vi "Printing Loop XYZ.vi"(11 "Stage Actor in":refnum<class "Stage.lvclass">) -> (3 "data value reference":refnum<data-value>)   [LabVIEW 2018, in "Stage Actor.lvlib" / "Stage.lvclass"]
uses:
  Stage.lvclass
  C:/Program Files/National Instruments/LabVIEW 2018/vi.lib/MGI/Panel Manager/Panel Actor/Panel Actor/Panel Actor.lvclass
  C:/Program Files/National Instruments/LabVIEW 2018/vi.lib/ActorFramework/Actor/Actor.lvclass
  Print Type Def.ctl
  <vilib>/ActorFramework/Actor/Actor.lvclass/Actor.ctl
  Stage.lvclass/Stage.ctl
  ADM/Main Messages/Set Flow Msg/Set Flow Msg.lvclass/Set Flow Msg.ctl
  <vilib>/ActorFramework/Message Enqueuer/Message Enqueuer.lvclass/Message Enqueuer.ctl
  ea4cf82d-fce5-4455-9177-557e4ebb6024.vi
  <vilib>/ActorFramework/Message Enqueuer/Enqueue.vi
  ADM/Main Messages/Set Flow Msg/Set Flow Msg.lvclass
  C:/Program Files/National Instruments/LabVIEW 2018/vi.lib/ActorFramework/Message/Message.lvclass
  Stage Messages/End Print Msg/End Print Msg.lvclass
  <vilib>/ActorFramework/Message Priority Queue/Priority Enqueue.vi
  <vilib>/MGI/Panel Manager/Panel Actor/Panel Actor/Panel Actor.lvclass
  Stage Actor.lvlib
  <instrlib>/Zaber A Series/Zaber A Series.lvlib
  <vilib>/ActorFramework/Actor/Actor.lvclass
panel:
  in  "Print Cancelled":bool
  in  "Stop":bool
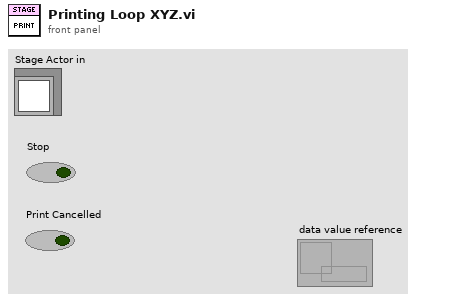
[diagram p1: front panel]
types:
  T1 = typedef "Stage Actor.lvlib/Print Type Def.ctl" = enum16{"Wait for Command", "Print Line", "End Print", "End"}
  T2 = cluster{"Current Tool":i16, "Speed":dbl, "Feeder State":bool, "Z":dbl, "XY":dbl[], "Theta Phi":dbl[]}
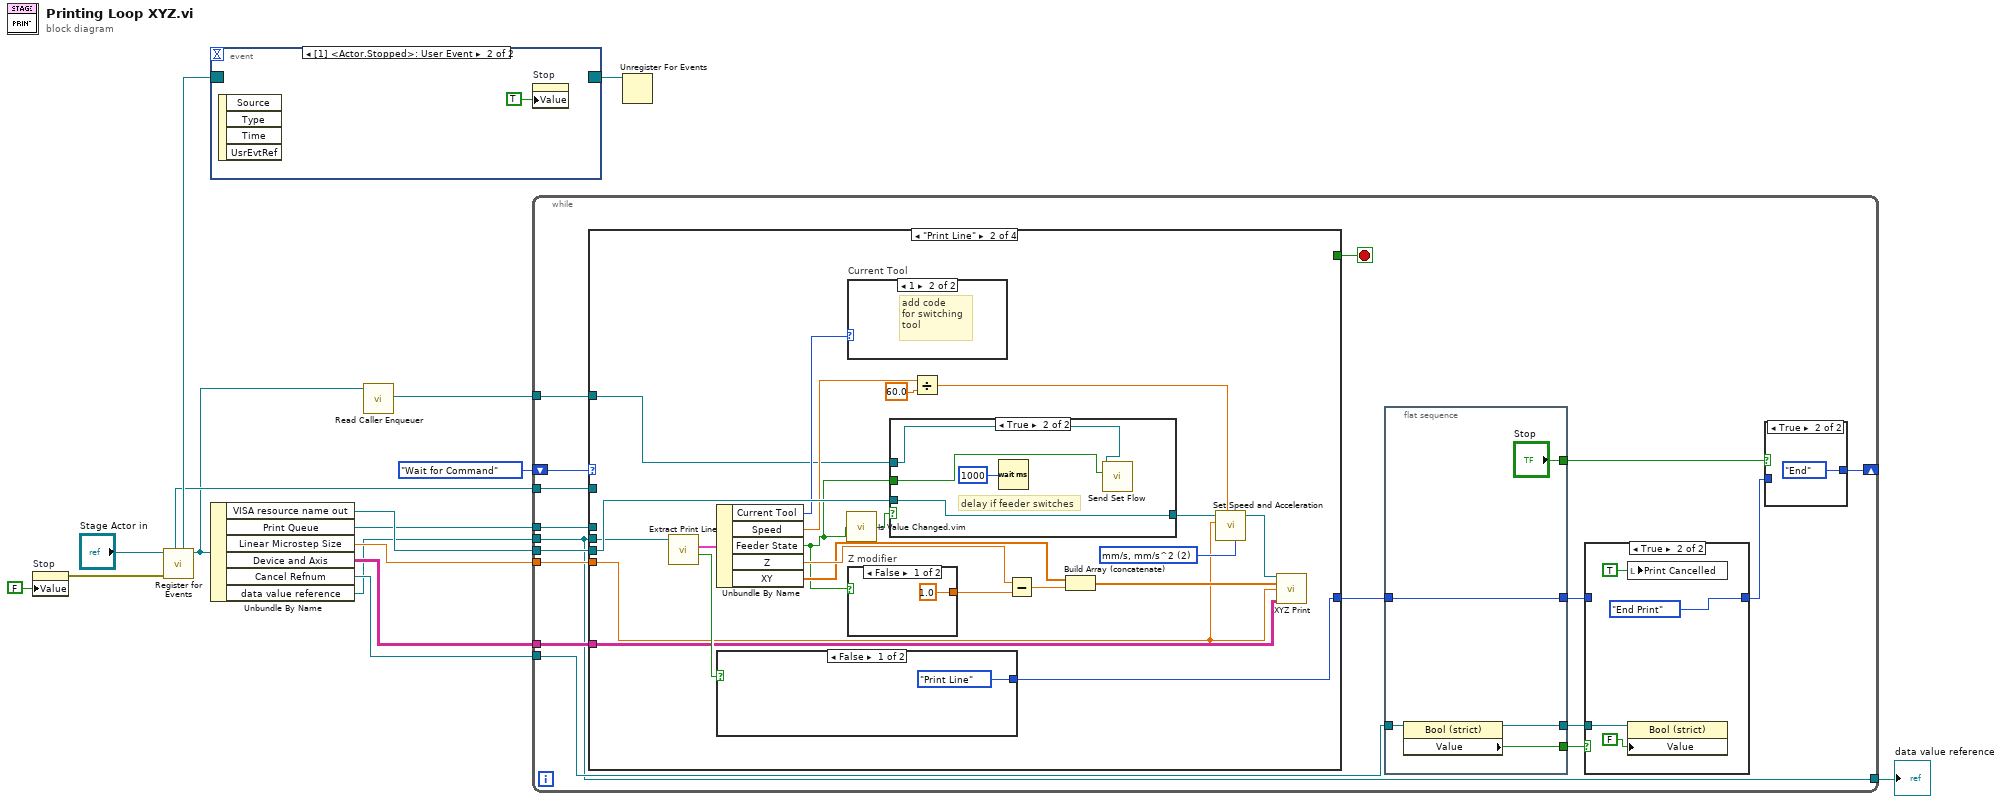
[diagram p0: block diagram]
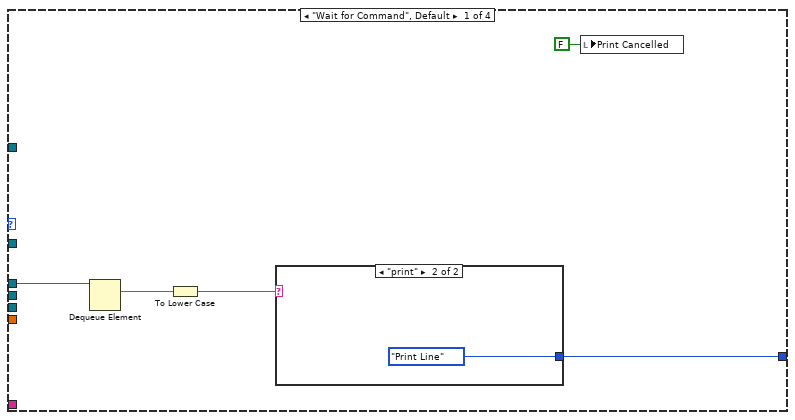
[diagram p4: hidden frame]
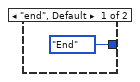
[diagram p5: hidden frame]
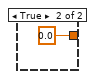
[diagram p6: hidden frame]
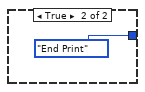
[diagram p7: hidden frame]
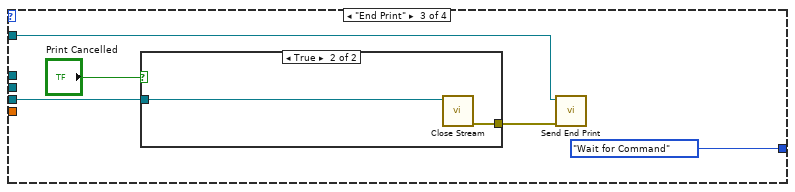
[diagram p10: hidden frame]
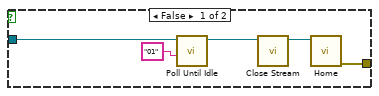
[diagram p11: hidden frame]
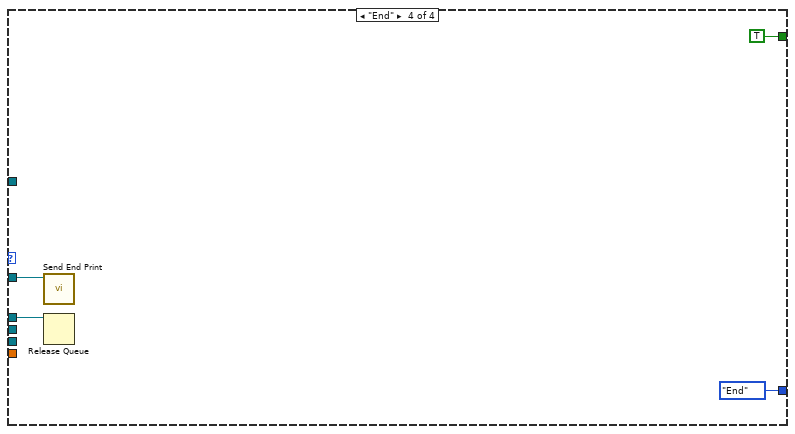
[diagram p12: hidden frame]
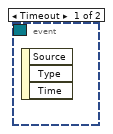
[diagram p13: hidden frame]
diagram:
  n1 = property on="Stop" class="Bool (strict)"("Value"=FALSE ("Stop")) -> (error out=w15:errorcluster)  [unwired: 2 in, 1 out]
  n2 = call <vilib>:"Register for Events.vi"("Error In"=w15, "Panel Actor in"="Stage Actor in") -> ("Panel Actor out"=w2:refnum<class "Stage.lvclass">, "Pnl Actor"=w16:refnum<event-registration>, "Self Enqueuer"=w5:refnum<class "Message Enqueuer.lvclass">)  [unwired: 6 in, 1 out]
  n3 = event shown="[1] <Actor.Stopped>: User Event" {
    selector: w16 -> [_ _]
    dyn-events: [_ _] -> w13
    timeout: _ -> [_ _]
    event Timeout {
      n4 = event-data() -> ()  [unwired: 1 in, 3 out]
    }
    event User Event {
      n5 = event-data() -> ()  [unwired: 1 in, 4 out]
      n6 = property on="Stop" class="Bool (strict)"("Value"=TRUE ("Stop")) -> ()  [unwired: 2 in, 2 out]
    }
  }
  n7 = Unbundle By Name(w2) -> ("VISA resource name out"=w10:refnum<visa-resource-name>, "Print Queue"=w9:refnum<queue>, "Linear Microstep Size"=w8:dbl, "Device and Axis"=w7:string[][], "Cancel Refnum"=w6:refnum<vi>, "data value reference"=w3:refnum<data-value>)
  n8 = call <vilib>:"Read Caller Enqueuer.vi"("Actor"=w2) -> ("Caller Enqueuer"=w1:refnum<class "Message Enqueuer.lvclass">)  [unwired: 10 in]
  n9 = while {
    shift-right: [w27] -> _
    shift-left: Print_Type_Def."Wait for Command" -> [w18]
    tunnel: w9 -> [w34]
    tunnel: w8 -> [w31]
    tunnel: w7 -> [w30]
    tunnel: w6 -> [w24]
    tunnel: w5 -> [w22]
    tunnel: w3 -> [w20]
    tunnel: [w20] -> w4
    tunnel: w10 -> [w21]
    tunnel: w1 -> [w19]
    stop <- w33 stop-if-true
    n10 = case shown="\"Print Line\"" w18 {
      tunnel: [w50 w65 Print_Type_Def."Wait for Command" Print_Type_Def."End"] -> w29
      tunnel: w21 -> [_ w74 w85 _]
      tunnel: w34 -> [w51 _ _ w100]
      tunnel: w20 -> [_ w67 _ _]
      tunnel: [_ _ _ TRUE] -> w33
      tunnel: w31 -> [_ w56 _ _]
      tunnel: w30 -> [_ w62 _ _]
      tunnel: w22 -> [_ _ w88 w97]
      tunnel: w19 -> [_ w55 _ _]
      frame "Wait for Command", Default {
        n11 = Dequeue Element(queue=w51) -> (element=w49:string)  [unwired: 2 in, 3 out]
        n12 = To Lower Case(string=w49) -> (all lower case string=w48:string)
        n13 = case shown="\"print\"" w48 {
          tunnel: [Print_Type_Def."End" Print_Type_Def."Print Line"] -> w50
          frame "end", Default {
          }
          frame "print" {
          }
        }
        n14 = local write "Print Cancelled"(FALSE ("Print Cancelled")) -> ()
      }
      frame "Print Line" {
        w60 = u16 2 items=["device units", "microns/s, microns/s^2", "mm/s, mm/s^2", "inches/s, inches/s^2", "degrees/s, degrees/s^2"] ("Units (0: data)")
        n15 = call "Extract Print Line.vi"("data value reference"=w67) -> ("End of Print?"=w66:bool, "Current Line"=w71:T2)  [unwired: 8 in, 1 out]
        n16 = Unbundle By Name(w71) -> ("Current Tool"=w69:i16, "Speed"=w70:dbl, "Feeder State"=w54:bool, "Z"=w64:dbl, "XY"=w59:dbl[])
        n17 = case shown="False" w66 {
          tunnel: [Print_Type_Def."Print Line" Print_Type_Def."End Print"] -> w65
          frame False {
          }
          frame True {
          }
        }
        n18 = call "Is Value Changed.vim"("value"=w54) -> ("changed or first call?"=w68:bool)
        n19 = case "Current Tool" shown="1" w69 {
          frame 0, Default {
          }
          frame 1 {
            # "add code\nfor switching \ntool"
          }
        }
        n20 = case "Z modifier" shown="False" w54 {
          tunnel: [1.0 0.0] -> w63
          frame False {
          }
          frame True {
          }
        }
        n21 = case shown="True" w68 {
          tunnel: w74 -> [w80 w84]
          tunnel: [w80 w84] -> w72
          tunnel: w55 -> [_ w82]
          tunnel: w54 -> [_ w81]
          frame False {
          }
          frame True {
            # "delay if feeder switches"
            n22 = Wait (ms)(milliseconds to wait=u32 1000) -> ()  [unwired: 1 out]
            n23 = call "Send Set Flow.vi"("State"=w81, "Message Enqueuer in"=w82) -> ()  [unwired: 8 in, 2 out]
          }
        }
        n24 = Divide(x=w70, y=60.0) -> (x/y=w61:dbl)
        n25 = Subtract(x=w64, y=w63) -> (x-y=w58:dbl)
        n26 = Build Array (concatenate)(w59, w58) -> (w57:dbl[])
        n27 = call <instrlib>:"Set Speed and Acceleration.vi"("Units (0: data)"=w60, "New Speed (0)"=w61, "Microstep Size (0)"=w56, "VISA resource name"=w72) -> ("VISA resource name out"=w75:refnum<visa-resource-name>)  [unwired: 6 in, 1 out]
        n28 = call "XYZ Print.vi"("VISA resource name"=w75, "XYZ"=w57, "Microstep Size (0)"=w56, "Device and Axis"=w62) -> ()  [unwired: 11 in, 1 out]
      }
      frame "End Print" {
        n29 = case shown="True" "Print Cancelled" {
          tunnel: w85 -> [w94 w95]
          tunnel: [w90 w96] -> w86
          frame False {
            n30 = call <instrlib>:"Poll Until Idle.vi"("Device and Axis"="01", "VISA resource name"=w94) -> ("VISA resource name out"=w93:refnum<visa-resource-name>)  [unwired: 8 in, 1 out]
            n31 = call <instrlib>:"Close Stream.vi"("VISA resource name"=w93) -> ("VISA resource name out"=w92:refnum<visa-resource-name>)  [unwired: 9 in, 1 out]
            n32 = call <instrlib>:"Home.vi"("VISA resource name"=w92) -> ("error out"=w90:errorcluster)  [unwired: 9 in, 1 out]
          }
          frame True {
            n33 = call <instrlib>:"Close Stream.vi"("VISA resource name"=w95) -> ("error out"=w96:errorcluster)  [unwired: 9 in, 1 out]
          }
        }
        n34 = call "Send End Print.vi"("error in (no error)"=w86, "Message Enqueuer in"=w88) -> ()  [unwired: 8 in, 2 out]
      }
      frame "End" {
        n35 = call "Send End Print.vi"("Message Enqueuer in"=w97) -> ()  [unwired: 9 in, 2 out]
        n36 = Release Queue(queue=w100) -> ()  [unwired: 2 in, 3 out]
      }
    }
    n37 = flat-sequence {
      tunnel: ["Stop"] -> w32
      tunnel: w29 -> [w43]
      tunnel: [w43] -> w26
      tunnel: [w40] -> w28
      tunnel: w24 -> [w42]
      tunnel: [w41] -> w23
      frame #0 {
        n38 = property class="Bool (strict)"(reference=w42) -> (reference out=w41:refnum<vi>, "Value"=w40:bool)  [unwired: 1 in, 1 out]
      }
    }
    n39 = case shown="True" w28 {
      tunnel: w26 -> [w35 _]
      tunnel: [w35 Print_Type_Def."End Print"] -> w25
      tunnel: w23 -> [_ w37]
      frame False {
      }
      frame True {
        n40 = local write "Print Cancelled"(TRUE ("Print Ended")) -> ()
        n41 = property class="Bool (strict)"(reference=w37, "Value"=FALSE) -> ()  [unwired: 1 in, 2 out]
      }
    }
    n42 = case shown="True" w32 {
      tunnel: w25 -> [w45 _]
      tunnel: [w45 Print_Type_Def."End"] -> w27
      frame False {
      }
      frame True {
      }
    }
  }
  "data value reference" <- w4
  n43 = Unregister For Events(event registration refnum=w13) -> ()  [unwired: 1 in, 1 out]
